vi "MBT_CreateLogEntry.vi"(10 "Array":string[](array[string]), 11 "MulticolumnListbox in":refnum<vi>) -> ()   [LabVIEW 2012, in "MBT_ModbusTester.lvlib"]
uses:
  MBT_ModbusTester.lvlib
  <vilib>/Utility/miscctls.llb/LVRowAndColumnUnsignedTypeDef.ctl
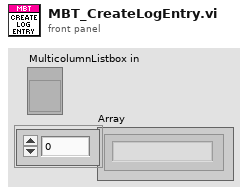
[diagram p1: front panel]
types:
  T1 = typedef "LVRowAndColumnUnsignedTypeDef.ctl" = cluster{"Row":u32, "Column":u32}
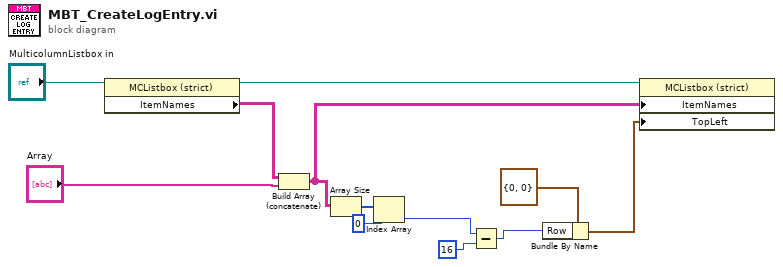
[diagram p0: block diagram]
diagram:
  n1 = property class="MCListbox (strict)"(reference="MulticolumnListbox in") -> (reference out=w9:refnum<vi>, "ItemNames"=w12:string[][])  [unwired: 1 in, 1 out]
  n2 = Build Array (concatenate)(w12, "Array") -> (w8:string[][])
  n3 = Array Size(array=w8) -> (size(s)=w7:i32[])
  n4 = Index Array(array=w7, index=0) -> (element=w2:i32)
  n5 = Subtract(x=w2, y=u32 16) -> (x-y=w1:u32)
  n6 = Bundle By Name(cluster=T1 {"Row"=0, "Column"=0} ("Top Left Visible Cell"), "Row"=w1) -> (w4:T1)
  n7 = property class="MCListbox (strict)"(reference=w9, "ItemNames"=w8, "TopLeft"=w4) -> ()  [unwired: 1 in, 2 out]
